vi "Parse node.vi"(10 "node paths":string[](array[string])=["oscs/0/freq", "sigouts/0/on", "demods/0/timeconstant", "demods/0/harmonic", "demods/0/rate", "sigins/0/range"]) -> (1 "parameters Array":string[](array[string]), 2 "No. Array":string[](array[string]), 3 "resource Array":string[](array[string]))   [LabVIEW 2016]
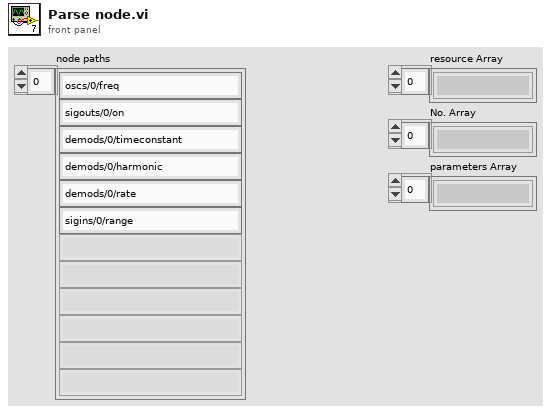
[diagram p1: front panel]
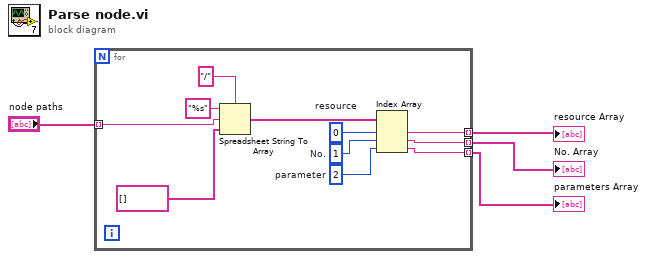
[diagram p0: block diagram]
diagram:
  n1 = for {
    tunnel: "node paths" -> [w14] mode=indexing
    tunnel: [w7] -> w3 mode=indexing
    tunnel: [w6] -> w2 mode=indexing
    tunnel: [w5] -> w1 mode=indexing
    w8 = 2  # parameter
    w9 = 1  # No.
    w10 = 0  # resource
    n2 = Spreadsheet String To Array(delimiter (Tab)="/", format string="%s", spreadsheet string=w14, array type (2D Dbl)=string[] []) -> (array=w11:string[])
    n3 = Index Array(array=w11, index #1=w10, index #2=w9, index #3=w8) -> (element #1=w7:string, element #2=w6:string, element #3=w5:string)
  }
  "resource Array" <- w3
  "No. Array" <- w2
  "parameters Array" <- w1
